vi "Auto Drive.vi"(6 "Reinitialize":bool, 8 "Strafe target":dbl, 9 "Heading target":dbl, 10 "Y target":dbl) -> (0 "X out":dbl, 1 "Strafe out":dbl, 2 "Y out":dbl)   [LabVIEW 2014]
uses:
  Common Code/Change Detect Boolean.vi
  Common Code/Change Detect Double.vi
panel:
  in  "Max Stop Speed":dbl
  in  "Distance Stop Treshold":dbl
  in  "omni?":bool
  in  "PID Params":T1={"X Dist"={"PID gains"={"proportional gain (Kc)"=1.0, "integral time (Ti, min)"=0.0, "derivative time (Td, min)"=0.0}, "output range"={"output high"=1.0, "output low"=-1.0}}, "Y Dist"={"PID gains"={"proportional gain (Kc)"=1.0, "integral time (Ti, min)"=0.0, "derivative time (Td, min)"=0.0}, "output range"={"output high"=1.0, "output low"=-1.0}}} {"Y Dist"."output range"."output low" format="%.2f"; "Y Dist"."output range"."output high" format="%.2f"; "Y Dist"."PID gains"."derivative time (Td, min)" format="%.3f"; "Y Dist"."PID gains"."integral time (Ti, min)" format="%.3f"; "Y Dist"."PID gains"."proportional gain (Kc)" format="%.3f"; "X Dist"."output range"."output low" format="%.2f"; "X Dist"."output range"."output high" format="%.2f"; "X Dist"."PID gains"."derivative time (Td, min)" format="%.3f"; "X Dist"."PID gains"."integral time (Ti, min)" format="%.3f"; "X Dist"."PID gains"."proportional gain (Kc)" format="%.3f"}
  out "isFinished":bool
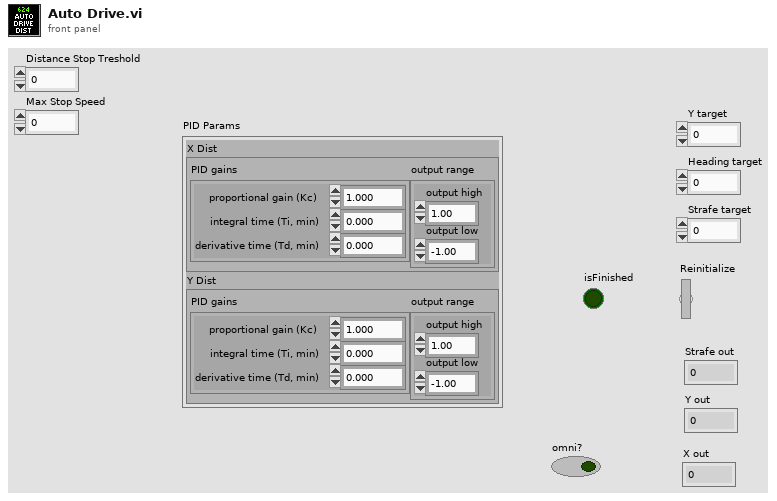
[diagram p1: front panel]
types:
  T1 = cluster{"X Dist":cluster{"PID gains":cluster{"proportional gain (Kc)":dbl, "integral time (Ti, min)":dbl, "derivative time (Td, min)":dbl}, "output range":cluster{"output high":dbl, "output low":dbl}}, "Y Dist":cluster{"PID gains":cluster{"proportional gain (Kc)":dbl, "integral time (Ti, min)":dbl, "derivative time (Td, min)":dbl}, "output range":cluster{"output high":dbl, "output low":dbl}}}
  T2 = typedef "Encoder Data.ctl" = cluster{"Avg Distance L/R":dbl, "Avg Speed L/R":dbl, "Left":T3, "Right":T3, "Omni":T3}
  T3 = typedef "Single Encoder Data.ctl" = cluster{"Distance":dbl, "Speed":dbl, "Ticks":dbl}
  T4 = cluster{"PID gains":cluster{"proportional gain (Kc)":dbl, "integral time (Ti, min)":dbl, "derivative time (Td, min)":dbl}, "output range":cluster{"output high":dbl, "output low":dbl}}
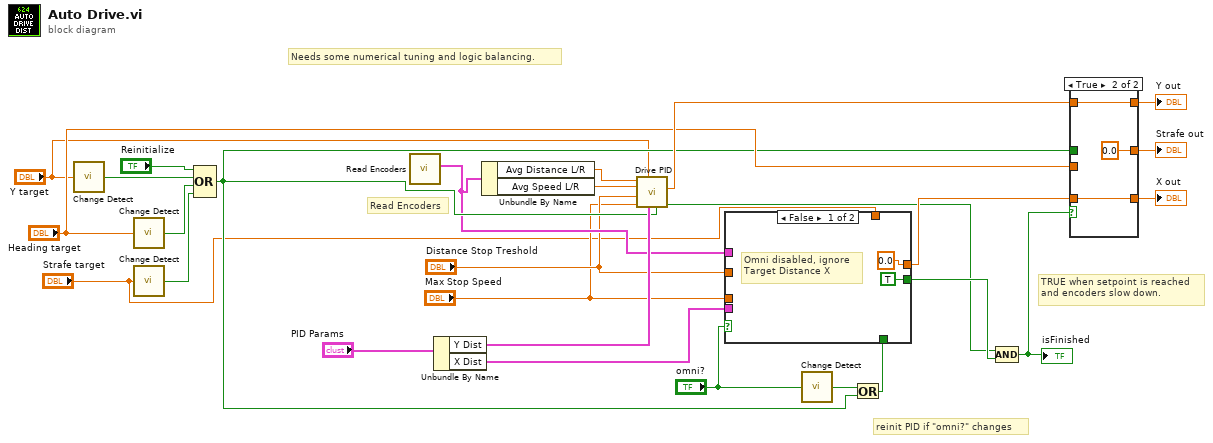
[diagram p0: block diagram]
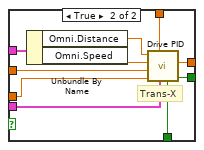
[diagram p2: hidden frame]
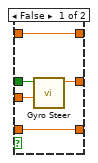
[diagram p3: hidden frame]
diagram:
  # "Needs some numerical tuning and logic balancing."
  # "reinit PID if \"omni?\" changes"
  # "Read Encoders"
  # "TRUE when setpoint is reached\nand encoders slow down."
  n1 = call-poly "Change Detect.vi"("In"="Y target") -> ("Changed?"=w27:bool)
  n2 = call-poly "Change Detect.vi"("In"="Heading target") -> ("Changed?"=w26:bool)
  n3 = call-poly "Change Detect.vi"("In"="Strafe target") -> ("Changed?"=w25:bool)
  n4 = Compound Arithmetic op=OR("Reinitialize", w27, w26, w25) -> (w8:bool)
  n5 = call "Read Encoders.vi"() -> ("Encoder Data"=w6:T2)  [unwired: 11 in]
  n6 = Unbundle By Name("PID Params") -> ("Y Dist"=w20:T4, "X Dist"=w19:T4)
  n7 = Unbundle By Name(w6) -> ("Avg Distance L/R"=w4:dbl, "Avg Speed L/R"=w5:dbl)
  n8 = call "Drive PID.vi"("reinitialize? (F)"=w8, "PID Params"=w20, "Setpoint"="Y target", "Max Stop Speed"="Max Stop Speed", "Distance Stop Threshold"="Distance Stop Treshold", "Current Speed"=w5, "Current Distance"=w4) -> ("Finished"=w10:bool, "output"=w13:dbl)  [unwired: 3 in]
  n9 = call-poly "Change Detect.vi"("In"="omni?") -> ("Changed?"=w16:bool)
  n10 = Or(x=w16, y=w8) -> (x .or. y?=w15:bool)
  n11 = case shown="False" "omni?" {
    tunnel: w19 -> [_ w39]
    tunnel: [0.0 ("output") w37] -> w17
    tunnel: [TRUE ("Finished") w36] -> w11
    tunnel: "Strafe target" -> [_ w35]
    tunnel: w15 -> [_ w34]
    tunnel: w6 -> [_ w32]
    tunnel: "Distance Stop Treshold" -> [_ w31]
    tunnel: "Max Stop Speed" -> [_ w30]
    frame False {
      # "Omni disabled, ignore\nTarget Distance X"
    }
    frame True {
      # "Trans-X"
      n12 = Unbundle By Name(w32) -> ("Omni.Distance"=w33:dbl, "Omni.Speed"=w38:dbl)
      n13 = call "Drive PID.vi"("reinitialize? (F)"=w34, "PID Params"=w39, "Setpoint"=w35, "Max Stop Speed"=w30, "Distance Stop Threshold"=w31, "Current Speed"=w38, "Current Distance"=w33) -> ("Finished"=w36:bool, "output"=w37:dbl)  [unwired: 3 in]
    }
  }
  n14 = Compound Arithmetic op=AND(w10, w11) -> (w12:bool)
  "isFinished" <- w12
  n15 = case shown="True" w12 {
    tunnel: "Heading target" -> [w42 _]
    tunnel: w8 -> [w41 _]
    tunnel: w13 -> [w44 w46]
    tunnel: [w40 0.0 ("Steering Out")] -> w23
    tunnel: [w44 w46] -> w22
    tunnel: [w43 w45] -> w18
    tunnel: w17 -> [w43 w45]
    frame False {
      n16 = call "Gyro Steer.vi"("Target Angle"=w42, "Changed?"=w41) -> ("X out"=w40:dbl)  [unwired: 9 in]
    }
    frame True {
    }
  }
  "Strafe out" <- w23
  "Y out" <- w22
  "X out" <- w18
